vi "Read DataTable.vi"(8 "error in (no error)":errorcluster, 11 "DataTable in":refnum<class "DataTable.lvclass">) -> (0 "error out":errorcluster, 2 "DataTable":refnum<k24>, 3 "DataTable out":refnum<class "DataTable.lvclass">)   [LabVIEW 2014, in "DataTable.lvclass"]
uses:
  DataTable.lvclass
  System.Data
  DataTable.lvclass/DataTable.ctl
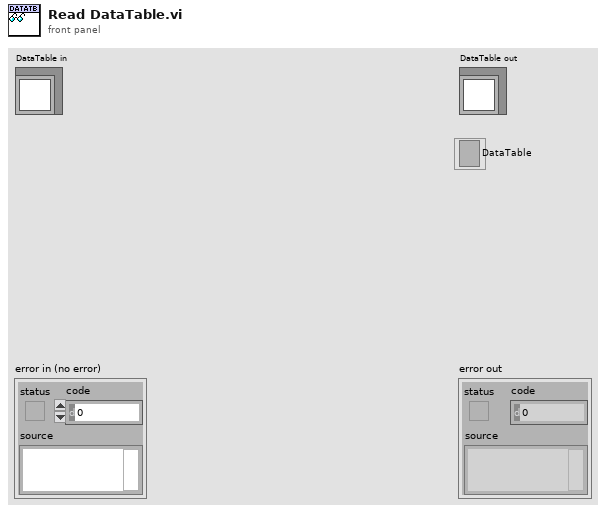
[diagram p1: front panel]
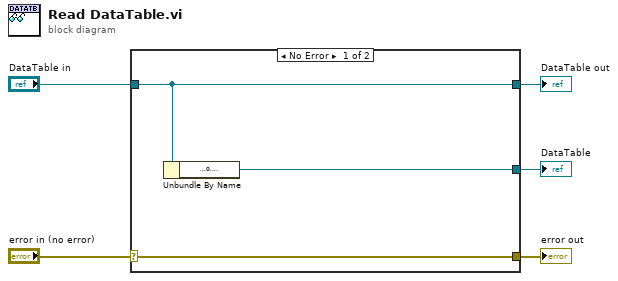
[diagram p0: block diagram]
diagram:
  n1 = case shown="No Error" "error in (no error)" {
    selector: "error in (no error)" -> [w8 w9]
    tunnel: [w8 w9] -> w4
    tunnel: [w7 w10] -> w2
    tunnel: "DataTable in" -> [w7 w10]
    tunnel: [w6 _] -> w1
    frame No Error {
      n2 = Unbundle By Name(w7) -> ("DataTable"=w6:refnum<k24>)
    }
    frame Error {
    }
  }
  "error out" <- w4
  "DataTable out" <- w2
  "DataTable" <- w1
